vi "Configure FFT Characteristics.vi"(0 "VISA resource name":refnum<visa-resource-name>, 1 "Enable FFT Display (T: Enable)":bool=TRUE, 2 "FFT Vertical Offset (0.0)":dbl, 3 "FFT Vertical Range (8.0 V)":dbl=8.0, 5 "FFT Center Frequency (50000.0 Hz)":dbl=50000.0, 7 "FFT Frequency Span (100000.0 Hz)":dbl=100000.0, 9 "FFT Reference Level (0.0)":dbl, 11 "error in (no error)":errorcluster, 12 "FFT Vertical Scale Units (0: dB)":i32(ring) items=["dB", "VRMS"], 13 "FFT Vertical Scale (10.0)":dbl=10.0) -> (4 "VISA resource name out":refnum<visa-resource-name>, 15 "error out":errorcluster)   [LabVIEW 2017, in "Agilent 2000 3000 X-Series.lvlib"]
doc: "Configures the characteristics of the FFT function.\n\nNotes:\nOnly applicable for 3000 T, 3000G, and 1000 Series. \nThe FFT subsystem controls the FFT function in the oscilloscope."
uses:
  Agilent 2000 3000 X-Series.lvlib
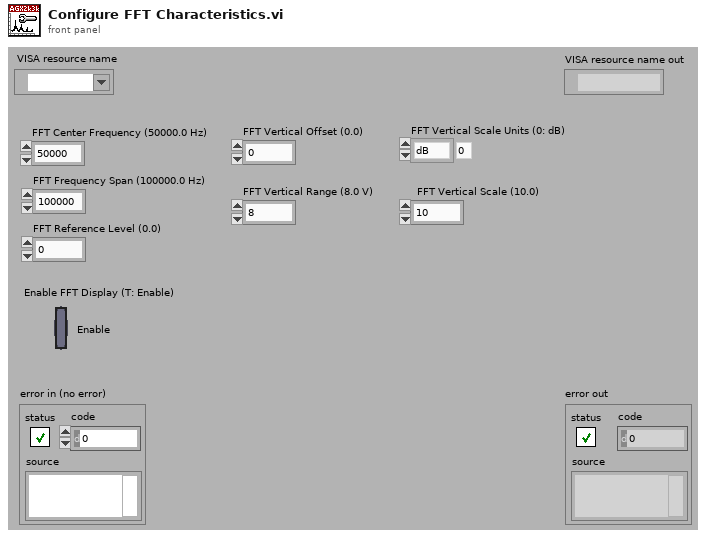
[diagram p1: front panel]
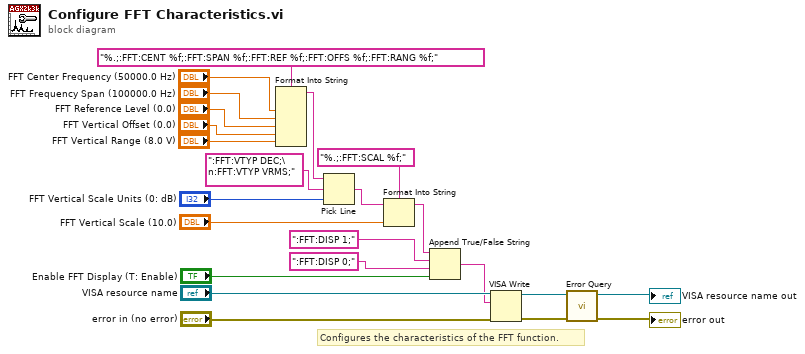
[diagram p0: block diagram]
diagram:
  # "Configures the characteristics of the FFT function."
  n1 = Format Into String(format string="%.;:FFT:CENT %f;:FFT:SPAN %f;:FFT:REF %f;:FFT:OFFS %f;:FFT:RANG %f;", "FFT Center Frequency (50000.0 Hz)", "FFT Frequency Span (100000.0 Hz)", "FFT Reference Level (0.0)", "FFT Vertical Offset (0.0)", "FFT Vertical Range (8.0 V)") -> (resulting string=w11:string)  [unwired: 2 in, 1 out]
  n2 = Pick Line(string ("")=w11, multi-line string=":FFT:VTYP DEC;\n:FFT:VTYP VRMS;", line index="FFT Vertical Scale Units (0: dB)") -> (output string=w8:string)
  n3 = Format Into String(format string="%.;:FFT:SCAL %f;", initial string=w8, "FFT Vertical Scale (10.0)") -> (resulting string=w5:string)  [unwired: 1 in, 1 out]
  n4 = Append True/False String(1:"Enable FFT Display (T: Enable)", 2:":FFT:DISP 0;" ("false string"), 3:":FFT:DISP 1;" ("true string"), 4:w5) -> (0:w1:string)
  n5 = VISA Write(VISA resource name="VISA resource name", write buffer=w1, error in (no error)="error in (no error)") -> (VISA resource name out=w22:refnum<visa-resource-name>, error out=w21:errorcluster)  [unwired: 1 out]
  n6 = call "Error Query.vi"("error in (no error)"=w21, "VISA resource name"=w22) -> ("error out"=→"error out":errorcluster, "VISA resource name out"=→"VISA resource name out":refnum<visa-resource-name>)  [unwired: 8 out]
